vi "Update Protocol UI Controls.vi"(9 "Frame Sync Clock Control":T5, 10 "PCM Data Configuration":T1, 11 "Control references":refnum<vi>[](array[refnum])) -> ()   [LabVIEW 2021]
uses:
  <vilib>/PDM Acquisition Toolkit/shared/controls/PCM Frame Sync Control.ctl
  <vilib>/PDM Acquisition Toolkit/shared/controls/Digital Edge.ctl
  <vilib>/PDM Acquisition Toolkit/shared/controls/PCM Data Format Configuration.ctl
  <vilib>/PDM Acquisition Toolkit/shared/controls/PCM Bit Endianness.ctl
  <vilib>/PDM Acquisition Toolkit/shared/controls/PCM Data Justification.ctl
  <vilib>/PDM Acquisition Toolkit/shared/PDM Shared.lvlib
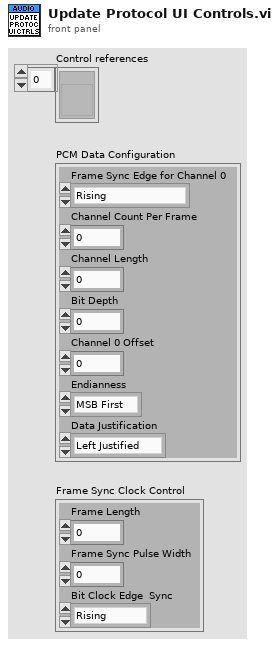
[diagram p1: front panel]
types:
  T1 = typedef "PDM Shared.lvlib/PCM Data Format Configuration.ctl" = cluster{"Frame Sync Edge for Channel 0":T2, "Channel Count Per Frame":u8, "Channel Length":u16, "Bit Depth":u8, "Channel 0 Offset":u16, "Endianness":T3, "Data Justification":T4}
  T2 = typedef "PDM Shared.lvlib/Digital Edge.ctl" = enum8{"Rising", "Falling"}
  T3 = typedef "PDM Shared.lvlib/PCM Bit Endianness.ctl" = enum16{"MSB First", "LSB First"}
  T4 = typedef "PDM Shared.lvlib/PCM Data Justification.ctl" = enum16{"Left Justified", "Right Justified"}
  T5 = typedef "PDM Shared.lvlib/PCM Frame Sync Control.ctl" = cluster{"Frame Length":u16, "Frame Sync Pulse Width":u16, "Bit Clock Edge  Sync":T2}
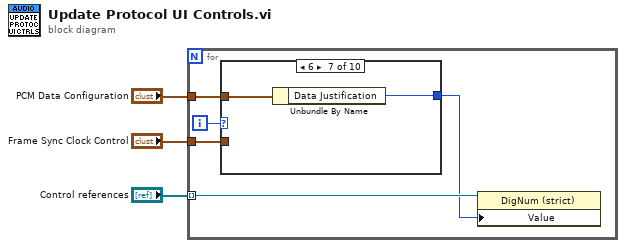
[diagram p0: block diagram]
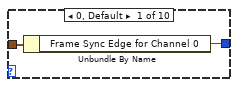
[diagram p2: hidden frame]
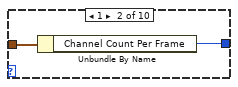
[diagram p3: hidden frame]
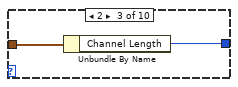
[diagram p4: hidden frame]
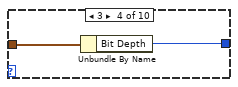
[diagram p5: hidden frame]
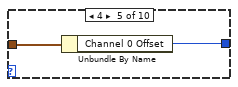
[diagram p6: hidden frame]
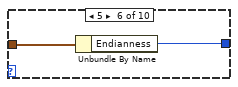
[diagram p7: hidden frame]
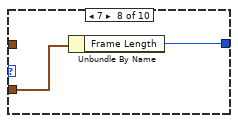
[diagram p8: hidden frame]
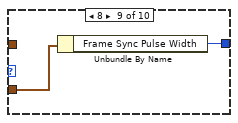
[diagram p9: hidden frame]
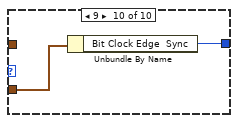
[diagram p10: hidden frame]
diagram:
  n1 = for {
    tunnel: "Control references" -> [w8] mode=indexing
    tunnel: "PCM Data Configuration" -> [w6]
    tunnel: "Frame Sync Clock Control" -> [w4]
    i -> [w7]
    n2 = case shown="6" w7 {
      tunnel: w6 -> [w10 w12 w14 w16 w18 w20 w22 _ _ _]
      tunnel: [w9 w11 w13 w15 w17 w19 w21 w24 w26 w28] -> w5
      tunnel: w4 -> [_ _ _ _ _ _ _ w23 w25 w27]
      frame 0, Default {
        n3 = Unbundle By Name(w10) -> ("Frame Sync Edge for Channel 0"=w9:T2)
      }
      frame 1 {
        n4 = Unbundle By Name(w12) -> ("Channel Count Per Frame"=w11:u8)
      }
      frame 2 {
        n5 = Unbundle By Name(w14) -> ("Channel Length"=w13:u16)
      }
      frame 3 {
        n6 = Unbundle By Name(w16) -> ("Bit Depth"=w15:u8)
      }
      frame 4 {
        n7 = Unbundle By Name(w18) -> ("Channel 0 Offset"=w17:u16)
      }
      frame 5 {
        n8 = Unbundle By Name(w20) -> ("Endianness"=w19:T3)
      }
      frame 6 {
        n9 = Unbundle By Name(w22) -> ("Data Justification"=w21:T4)
      }
      frame 7 {
        n10 = Unbundle By Name(w23) -> ("Frame Length"=w24:u16)
      }
      frame 8 {
        n11 = Unbundle By Name(w25) -> ("Frame Sync Pulse Width"=w26:u16)
      }
      frame 9 {
        n12 = Unbundle By Name(w27) -> ("Bit Clock Edge  Sync"=w28:T2)
      }
    }
    n13 = property class="DigNum (strict)"(reference=w8, "Value"=w5) -> ()  [unwired: 1 in, 2 out]
  }
